vi "DT3120_StartPassThru.vi"(8 "error in (no error)":errorcluster, 11 "DevId":i32) -> (0 "error out":errorcluster, 3 "DevId (dup)":i32)   [LabVIEW 2009]
uses:
  olfg32.dll
panel:
  in  "CurDevCaps":T1
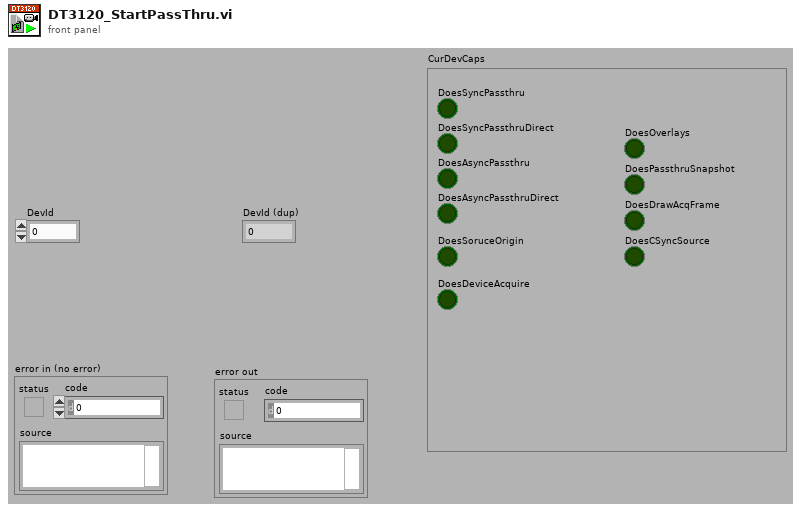
[diagram p1: front panel]
types:
  T1 = cluster{"DoesSyncPassthru":bool, "DoesSyncPassthruDirect":bool, "DoesAsyncPassthru":bool, "DoesAsyncPassthruDirect":bool, "DoesSoruceOrigin":bool, "DoesDeviceAcquire":bool, "DoesOverlays":bool, "DoesPassthruSnapshot":bool, "DoesDrawAcqFrame":bool, "DoesCSyncSource":bool}
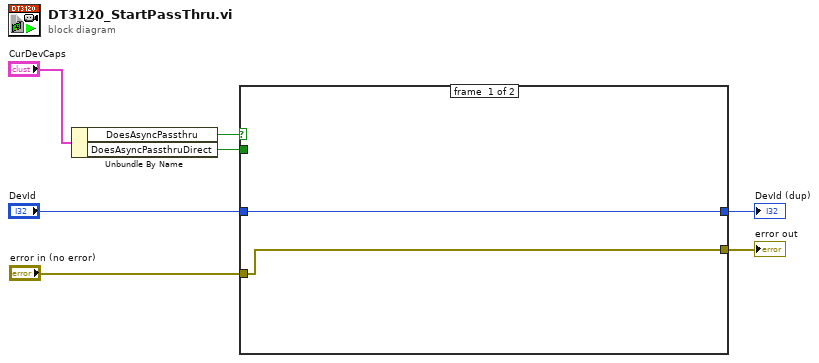
[diagram p0: block diagram]
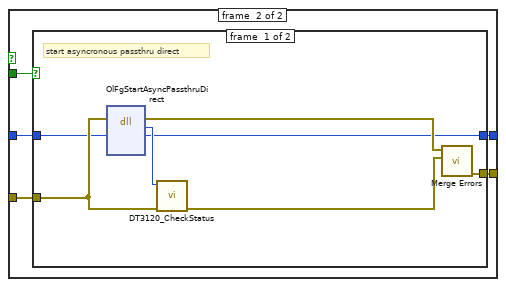
[diagram p2: hidden frame]
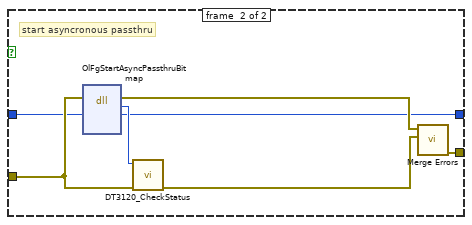
[diagram p3: hidden frame]
diagram:
  n1 = Unbundle By Name("CurDevCaps") -> ("DoesAsyncPassthru"=w2:bool, "DoesAsyncPassthruDirect"=w1:bool)
  n2 = case shown="True" w2 {
    tunnel: [w8 w14] -> w7
    tunnel: "error in (no error)" -> [w8 w13]
    tunnel: "DevId" -> [w9 w12]
    tunnel: [w9 w11] -> w4
    tunnel: w1 -> [_ w10]
    frame #0 {
    }
    frame #1 {
      n3 = case shown="True" w10 {
        tunnel: [w21 w28] -> w14
        tunnel: w13 -> [w20 w27]
        tunnel: w12 -> [w17 w24]
        tunnel: [w15 w22] -> w11
        frame #0 {
          # "start asyncronous passthru direct"
          n4 = dll-call lib="C:/LabVIEW Programs/MT Scan/SubVIs/olfg32.dll" fn="OlFgStartAsyncPassthruDirect"(error in=w20, "DevId"=w17) -> (error out=w19:errorcluster, "Status"=w18:u32, "DevId"=w15:i32)  [unwired: 4 in, 3 out]
          n5 = call "DT3120_CheckStatus.vi"("error in"=w20, "Status"=w18) -> ("error out"=w16:errorcluster)  [unwired: 9 out]
          n6 = call <vilib>:"Merge Errors.vi"("error in 2 (no error)"=w16, "error in 1 (no error)"=w19) -> ("error out"=w21:errorcluster)  [unwired: 2 in, 3 out]
        }
        frame #1 {
          # "start asyncronous passthru"
          n7 = dll-call lib="C:/LabVIEW Programs/MT Scan/SubVIs/olfg32.dll" fn="OlFgStartAsyncPassthruBitmap"(error in=w27, "DevId"=w24) -> (error out=w26:errorcluster, "Status"=w25:u32, "DevId"=w22:i32)  [unwired: 4 in, 3 out]
          n8 = call "DT3120_CheckStatus.vi"("error in"=w27, "Status"=w25) -> ("error out"=w23:errorcluster)  [unwired: 9 out]
          n9 = call <vilib>:"Merge Errors.vi"("error in 2 (no error)"=w23, "error in 1 (no error)"=w26) -> ("error out"=w28:errorcluster)  [unwired: 2 in, 3 out]
        }
      }
    }
  }
  "error out" <- w7
  "DevId (dup)" <- w4
